vi "GetLoadedDevTree.vi"(8 "ErrorIn":errorcluster caption="Entrée d'erreur", 9 "TreeRefIn":refnum<vi>, 10 "LoadedInst":refnum<class "BaseDevice.lvclass">[](array[class]), 11 "AvailRessArray":string[][](array[string])) -> (0 "ErrorOut":errorcluster caption="Sortie d'erreur")   [LabVIEW 2019, in "BaseDevice.lvclass"]
uses:
  BaseDevice.lvclass
  BaseDevice.lvclass/BaseDevice.ctl
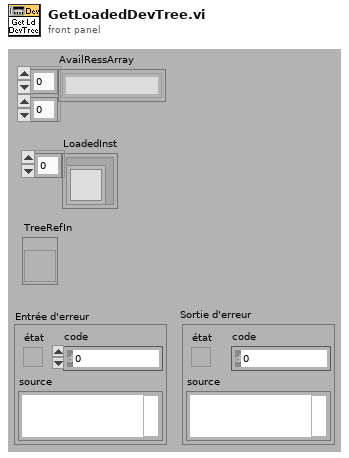
[diagram p1: front panel]
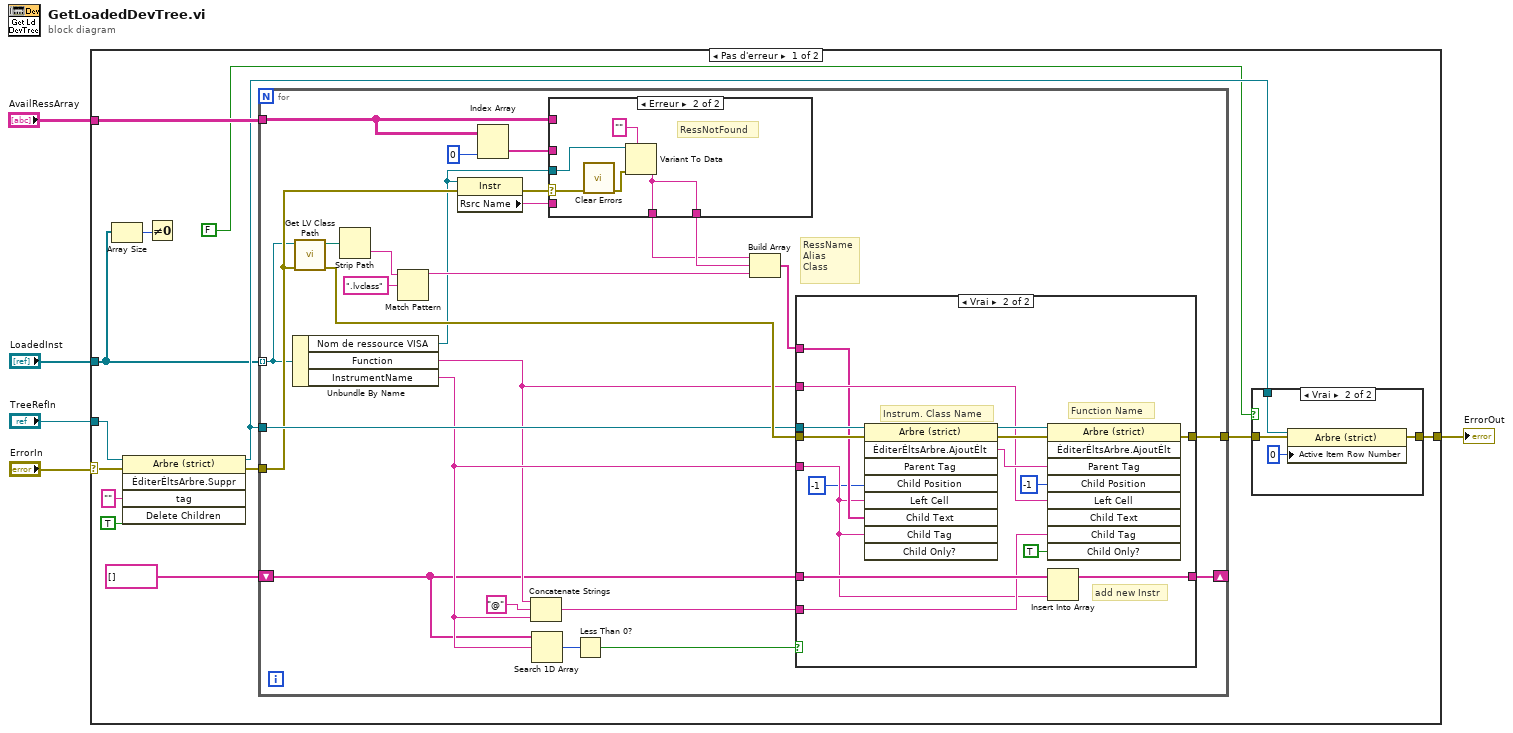
[diagram p0: block diagram]
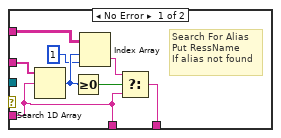
[diagram p3: hidden frame]
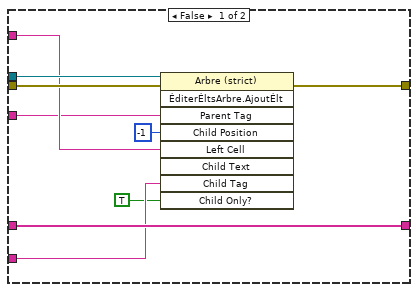
[diagram p4: hidden frame]
diagram:
  n1 = case shown="Pas d'erreur" "ErrorIn" {
    selector: "ErrorIn" -> [w15 w87]
    tunnel: "LoadedInst" -> [w8 _]
    tunnel: "AvailRessArray" -> [w18 _]
    tunnel: [w10 w87] -> w2
    tunnel: "TreeRefIn" -> [w16 _]
    frame No Error {
      n2 = Array Size(array=w8) -> (size(s)=w7:i32)
      n3 = invoke on="Nœud de méthode" class="Arbre (strict)" method="ÉditerÉltsArbre.Suppr"(reference=w16, error in=w15, "tag"="" ("Tag"), "Delete Children"=TRUE ("Supprimer les enfants ?")) -> (reference out=w9:refnum<vi>, error out=w14:errorcluster)  [unwired: 1 in, 3 out]
      n4 = Not Equal To 0?(x=w7) -> ()  [unwired: 1 out]
      n5 = for {
        tunnel: w8 -> [w25] mode=indexing
        tunnel: w18 -> [w44]
        shift-right: [w42] -> _
        shift-left: string[] [] -> [w24]
        tunnel: w14 -> [w31]
        tunnel: [w38] -> w11
        tunnel: w9 -> [w37]
        # "RessName\nAlias\nClass"
        n6 = Unbundle By Name(w25) -> ("Nom de ressource VISA"=w29:refnum<visa-resource-name>, "Function"=w26:string, "InstrumentName"=w27:string)
        n7 = call <vilib>:"Get LV Class Path.vi"("error in (no error)"=w31, "object"=w25) -> ("error out"=w39:errorcluster, "class path"=w49:path)  [unwired: 8 in]
        n8 = Strip Path(path=w49) -> (name=w47:string)  [unwired: 1 out]
        n9 = Match Pattern(string=w47, regular expression=".lvclass" ("expression régulière")) -> (before substring=w36:string)  [unwired: 1 in, 3 out]
        n10 = property class="Instr"(reference=w29, error in=w31) -> (error out=w30:errorcluster, "Rsrc Name"=w34:string)  [unwired: 1 out]
        n11 = Index Array(array=w44, index (col)=0 ("indice désactivé (col)")) -> (element=w45:string[])  [unwired: 1 in]
        n12 = Concatenate Strings(w26, "@" ("chaîne"), w27) -> (w32:string)
        n13 = Search 1D Array(1D array=w24, element=w27) -> (index of element=w41:i32)  [unwired: 1 in]
        n14 = case shown="Erreur" w30 {
          selector: w30 -> [_ w60]
          tunnel: w45 -> [w57 _]
          tunnel: w44 -> [w56 _]
          tunnel: [w52 w58] -> w35
          tunnel: w34 -> [w51 _]
          tunnel: w29 -> [_ w61]
          tunnel: [w51 w58] -> w28
          frame No Error {
            # "Search For Alias\nPut RessName \nIf alias not found"
            n15 = Search 1D Array(1D array=w57, element=w51) -> (index of element=w55:i32)  [unwired: 1 in]
            n16 = Greater Or Equal To 0?(x=w55) -> (x >= 0?=w53:bool)
            n17 = Index Array(array=w56, index (row)=w55, index (col)=1 ("indice désactivé (col)")) -> (element=w54:string)
            n18 = Select(t=w54, s=w53, f=w51) -> (s? t:f=w52:string)
          }
          frame Error {
            # "RessNotFound"
            n19 = call <vilib>:"Clear Errors.vi"("error in (no error)"=w60) -> ("error out"=w59:errorcluster)  [unwired: 5 in, 1 out]
            n20 = Variant To Data(error in=w59, type="" ("chaîne de données 2"), Variant=w61) -> (data=w58:string)  [unwired: 1 out]
          }
        }
        n21 = Less Than 0?(x=w41) -> (x < 0?=w40:bool)
        n22 = Build Array(w28, w35, w36) -> (w43:string[])
        n23 = case shown="Vrai" w40 {
          tunnel: w27 -> [w66 w74]
          tunnel: w26 -> [w67 w78]
          tunnel: w43 -> [_ w76]
          tunnel: w24 -> [w71 w84]
          tunnel: [w71 w83] -> w42
          tunnel: w39 -> [w70 w81]
          tunnel: [w69 w80] -> w38
          tunnel: w37 -> [w68 w79]
          tunnel: w32 -> [w65 w77]
          frame False {
            n24 = invoke on="Nœud de méthode" class="Arbre (strict)" method="ÉditerÉltsArbre.AjoutÉlt"(reference=w68, error in=w70, "Parent Tag"=w66, "Child Position"=-1 ("Position de l'enfant"), "Left Cell"=w67, "Child Tag"=w65, "Child Only?"=TRUE ("Enfant uniquement ?")) -> (error out=w69:errorcluster)  [unwired: 2 in, 8 out]
          }
          frame True {
            # "Function Name"
            # "Instrum. Class Name"
            # "add new Instr"
            n25 = invoke on="Nœud de méthode" class="Arbre (strict)" method="ÉditerÉltsArbre.AjoutÉlt"(reference=w79, error in=w81, "Child Position"=-1 ("Position de l'enfant"), "Left Cell"=w74, "Child Text"=w76, "Child Tag"=w74) -> (reference out=w85:refnum<vi>, error out=w86:errorcluster, "Edit Tree Items:Add Item"=w82:string)  [unwired: 3 in, 6 out]
            n26 = invoke on="Nœud de méthode" class="Arbre (strict)" method="ÉditerÉltsArbre.AjoutÉlt"(reference=w85, error in=w86, "Parent Tag"=w82, "Child Position"=-1 ("Position de l'enfant"), "Left Cell"=w78, "Child Tag"=w77, "Child Only?"=TRUE ("Enfant uniquement ?")) -> (error out=w80:errorcluster)  [unwired: 2 in, 8 out]
            n27 = Insert Into Array(array=w84, new element=w74) -> (w83:string[])  [unwired: 1 in]
          }
        }
      }
      n28 = case shown="Vrai" FALSE {
        tunnel: w11 -> [w19 w23]
        tunnel: [w19 w22] -> w10
        tunnel: w9 -> [_ w21]
        frame False {
          # "nothing loaded"
        }
        frame True {
          n29 = property class="Arbre (strict)"(reference=w21, error in=w23, "Active Item Row Number"=0 ("Élément actif : numéro de ligne")) -> (error out=w22:errorcluster)  [unwired: 1 out]
        }
      }
    }
    frame Error {
    }
  }
  "ErrorOut" <- w2
